vi "Update Arrival Time TIO.vi"(6 "Delay, ns":u32, 8 "error in":errorcluster, 9 "Number of Photons Counted":i32, 10 "Buffer In":i32[][](array[numeric]), 11 "Arrival Time Clusters":T1(array[cluster])) -> (0 "error out":errorcluster, 1 "Number of Photons Counted Out":i32, 2 "Buffer Out":i32[][](array[numeric]), 3 "Arrival Time Clusters":T1(array[cluster]), 4 "Dump Buffer":bool)   [LabVIEW 2009]
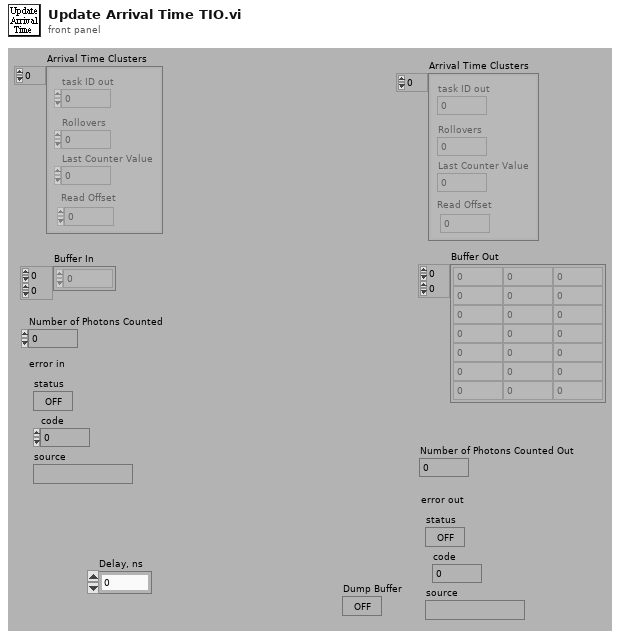
[diagram p1: front panel]
types:
  T1 = cluster{"task ID out":u32, "Rollovers":i32, "Last Counter Value":u32, "Read Offset":i32}[]
  T2 = cluster{"read/search mode":u32, "read/search offset":i32}
  T3 = cluster{"task ID out":u32, "Rollovers":i32, "Last Counter Value":u32, "Read Offset":i32}
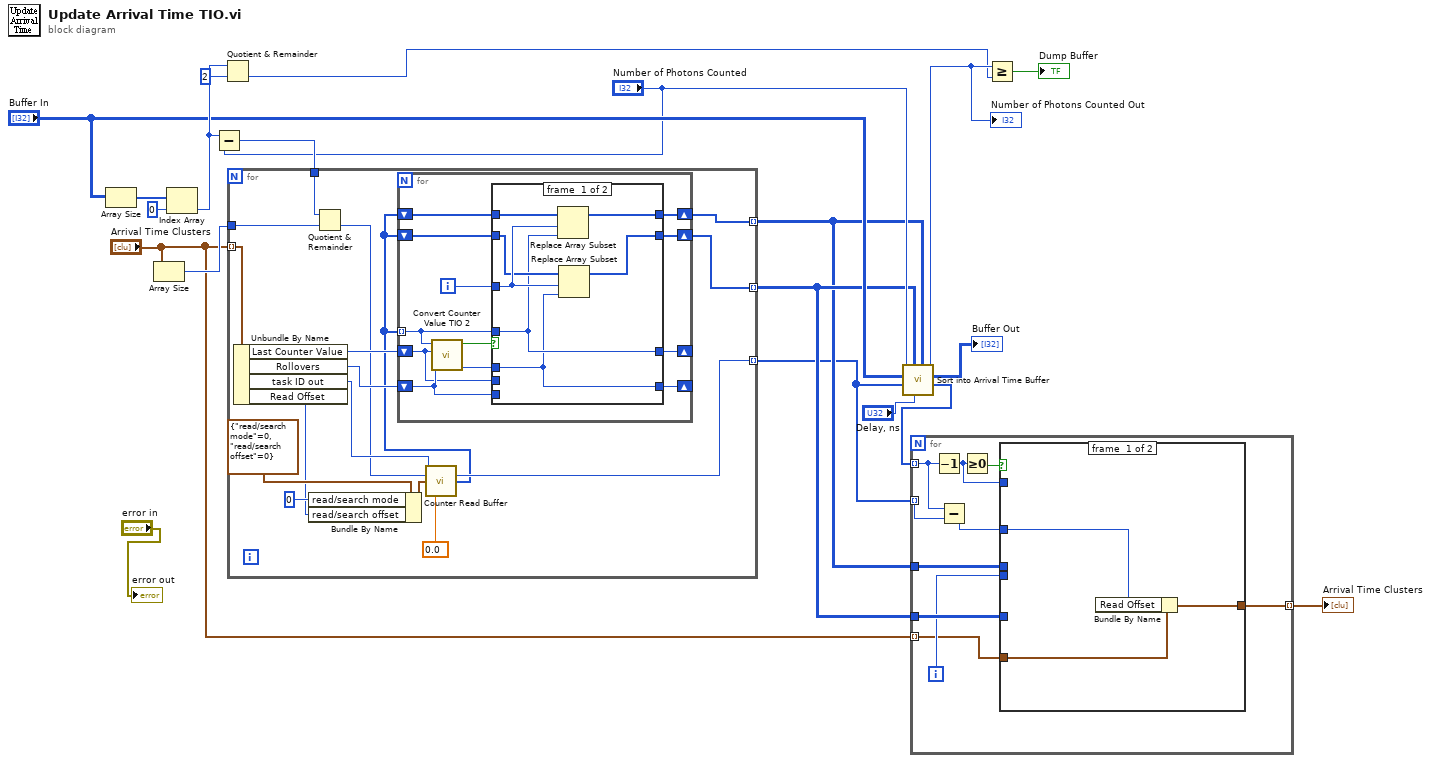
[diagram p0: block diagram]
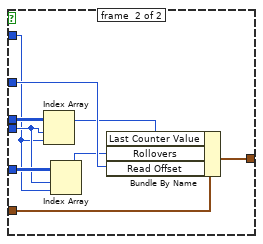
[diagram p2: hidden frame]
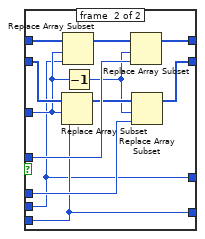
[diagram p3: hidden frame]
diagram:
  n1 = Array Size(array="Buffer In") -> (size(s)=w20:i32[])
  n2 = Array Size(array="Arrival Time Clusters") -> (size(s)=w18:i32)
  n3 = Index Array(array=w20, index=0 ("Index")) -> (element=w15:i32)
  n4 = Subtract(x=w15, y="Number of Photons Counted") -> (x-y=w17:i32)
  n5 = Quotient & Remainder(x=w15, y=2) -> (floor(x/y)=w13:i32)  [unwired: 1 out]
  n6 = for {
    tunnel: "Arrival Time Clusters" -> [w32] mode=indexing
    tunnel: w18 -> [w28]
    tunnel: [w22] -> w6 mode=indexing
    tunnel: [w21] -> w5 mode=indexing
    tunnel: [w27] -> w3 mode=indexing
    tunnel: w17 -> [w26]
    n7 = Unbundle By Name(w32) -> ("Last Counter Value"=w33:u32, "Rollovers"=w34:i32, "task ID out"=w35:u32, "Read Offset"=w24:i32)
    n8 = Bundle By Name(cluster=T2 {"read/search mode"=0, "read/search offset"=0} ("read/search position (from mark)"), "read/search mode"=u32 0, "read/search offset"=w24) -> (w31:T2)
    n9 = Quotient & Remainder(x=w26, y=w28) -> (floor(x/y)=w25:i32)  [unwired: 1 out]
    n10 = call <vilib>:"Counter Read Buffer.vi"("task ID"=w35, "number to read (-1: no change)"=w25, "read/search position (from mark)"=w31, "time limit (-1: no change)"=0.0) -> ("number read"=w27:u32, "binary data"=w23:u32[])  [unwired: 5 in, 5 out]
    n11 = for {
      tunnel: w23 -> [w44] mode=indexing
      shift-right: [w38] -> _
      shift-left: w33 -> [w39]
      shift-right: [w37] -> _
      shift-left: w34 -> [w40]
      shift-right: [w42] -> w21
      shift-left: w23 -> [w46]
      shift-right: [w41] -> w22
      shift-left: w23 -> [w45]
      i -> [w47]
      n12 = call "Convert Counter Value TIO 2.vi"("Rollovers"=w40, "Last Time of Arrival (counts)"=w39, "Time of Arrival (counts)"=w44) -> ("Rollovers Out"=w43:u32, "Reverse Order"=w48:bool)  [unwired: 7 in]
      n13 = case shown="True" w48 {
        tunnel: w47 -> [w54 w59]
        tunnel: w46 -> [w55 w63]
        tunnel: w45 -> [w53 w62]
        tunnel: w44 -> [w50 w67]
        tunnel: w43 -> [w49 w66]
        tunnel: [w52 w65] -> w42
        tunnel: [w51 w64] -> w41
        tunnel: w40 -> [_ w57]
        tunnel: w39 -> [_ w56]
        tunnel: [w50 w56] -> w38
        tunnel: [w49 w57] -> w37
        frame #0 {
          n14 = Replace Array Subset(array=w55, new element=w50, index=w54) -> (w52:u32[])
          n15 = Replace Array Subset(array=w53, new element=w49, index=w54) -> (w51:u32[])
        }
        frame #1 {
          n16 = Replace Array Subset(array=w62, new element=w57, index=w59) -> (w61:u32[])
          n17 = Replace Array Subset(array=w63, new element=w56, index=w59) -> (w60:u32[])
          n18 = Decrement(x=w59) -> (x-1=w58:i32)
          n19 = Replace Array Subset(array=w60, new element=w67, index=w58) -> (w65:u32[])
          n20 = Replace Array Subset(array=w61, new element=w66, index=w58) -> (w64:u32[])
        }
      }
    }
  }
  n21 = call "Sort into Arrival Time Buffer.vi"("Time Low"=w5, "Delay, ns"="Delay, ns", "Time High"=w6, "Size of Channel Arrays"=w3, "Buffer In"="Buffer In", "Number of Photons Counted In"="Number of Photons Counted") -> ("Index for Buffer"=w4:i32[], "Buffer Out"=→"Buffer Out":i32[][], "Number of Photons Counted Out"=w16:i32)  [unwired: 3 in]
  "Number of Photons Counted Out" <- w16
  n22 = for {
    tunnel: w4 -> [w69] mode=indexing
    tunnel: w5 -> [w77]
    tunnel: w6 -> [w76]
    tunnel: w3 -> [w68] mode=indexing
    tunnel: "Arrival Time Clusters" -> [w73] mode=indexing
    tunnel: [w72] -> w7 mode=indexing
    i -> [w75]
    n23 = Decrement(x=w69) -> (x-1=w74:i32)
    n24 = Subtract(x=w69, y=w68) -> (x-y=w70:u32)
    n25 = Greater Or Equal To 0?(x=w74) -> (x >= 0?=w71:bool)
    n26 = case shown="True" w71 {
      tunnel: w77 -> [_ w86]
      tunnel: w76 -> [_ w84]
      tunnel: w75 -> [_ w82]
      tunnel: w74 -> [_ w81]
      tunnel: w73 -> [w80 w89]
      tunnel: w70 -> [w79 w88]
      tunnel: [w78 w87] -> w72
      frame #0 {
        n27 = Bundle By Name(cluster=w80, "Read Offset"=w79) -> (w78:T3)
      }
      frame #1 {
        n28 = Index Array(array=w86, index (row)=w82, index (col)=w81) -> (element=w85:u32)
        n29 = Index Array(array=w84, index (row)=w82, index (col)=w81) -> (element=w83:u32)
        n30 = Bundle By Name(cluster=w89, "Last Counter Value"=w85, "Rollovers"=w83, "Read Offset"=w88) -> (w87:T3)
      }
    }
  }
  "Arrival Time Clusters" <- w7
  n31 = Greater Or Equal?(x=w16, y=w13) -> (x >= y?=→"Dump Buffer":bool)
  "error out" <- "error in"
